vi "采集的条码数组.vi"(9 "条码数量":i32, 10 "地址":string, 11 "开启条码?":bool) -> (1 "条码字符串":string, 2 "条码数组":string[](array[string]), 3 "料号":string[](array[string]))   [LabVIEW 2014]
panel:
  out "数组":string[](array[string])
  out "数据输出":string
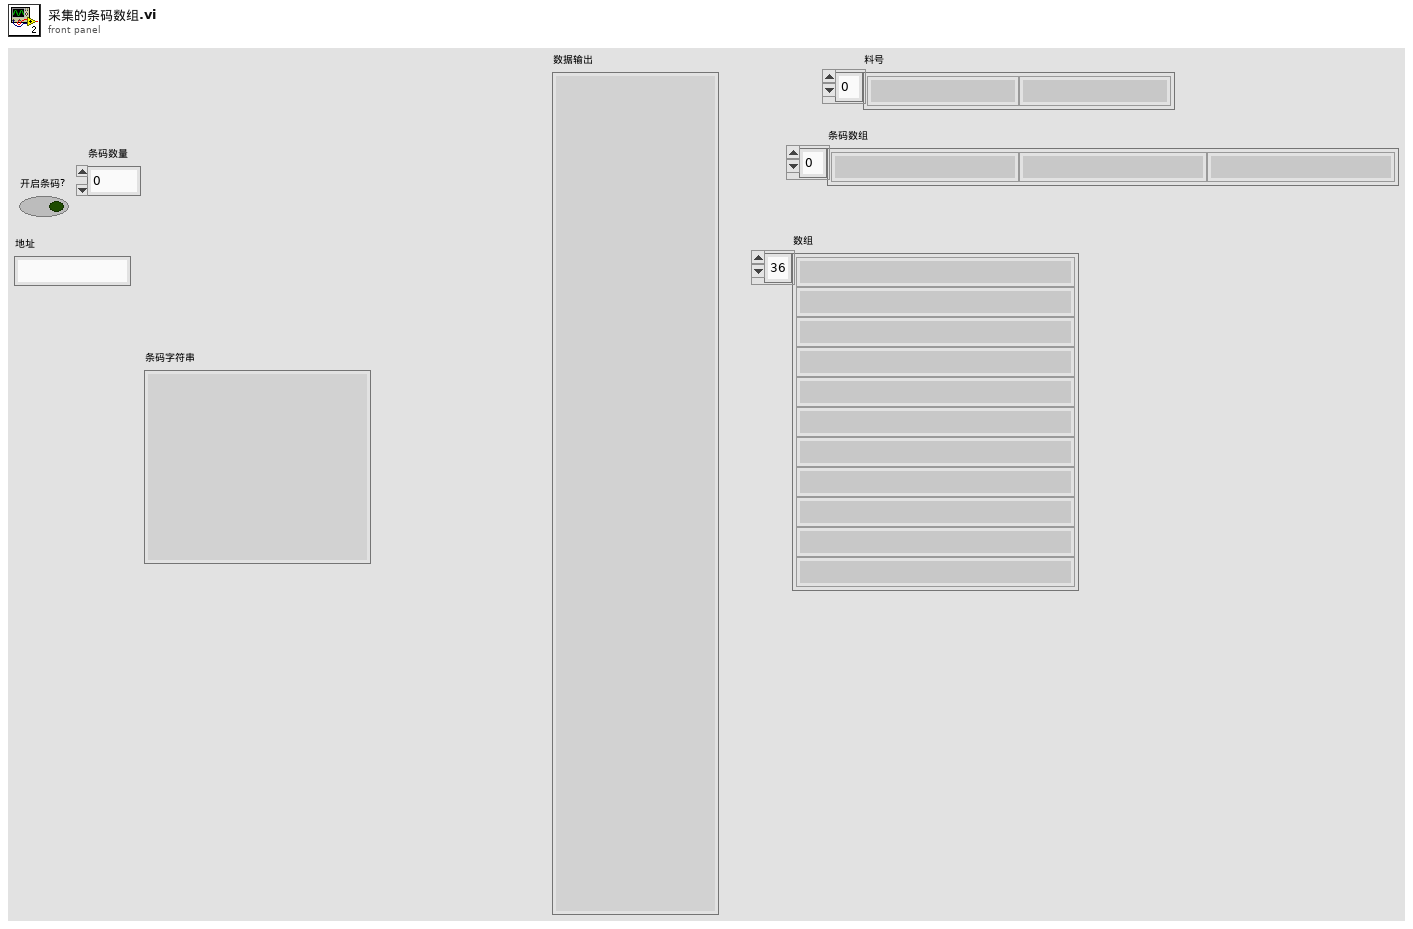
[diagram p1: front panel]
types:
  T1 = enum16{"Standard", "Buffered", "CRLF", "Immediate"}
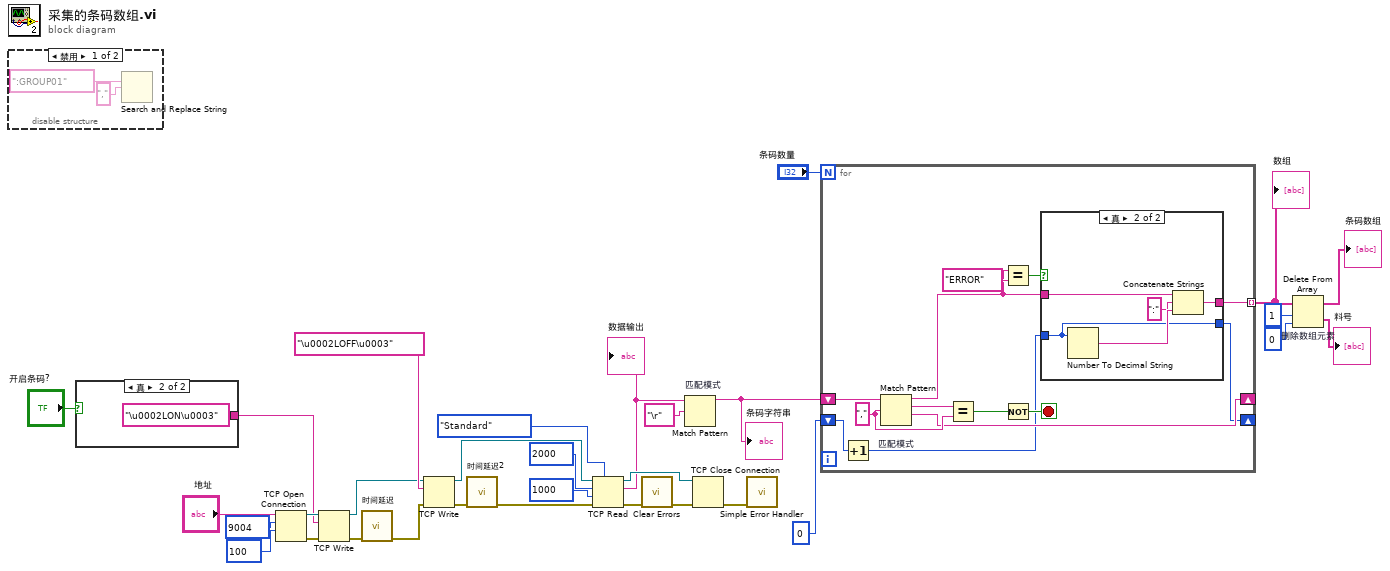
[diagram p0: block diagram]
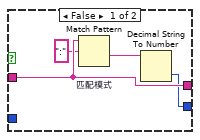
[diagram p3: hidden frame]
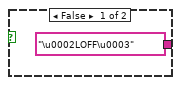
[diagram p4: hidden frame]
diagram:
  n1 = disable-structure shown="禁用" {
    frame Disabled {
      n2 = Search and Replace String ("搜索替换字符串")(search string=":GROUP01" ("正则表达式"), replace string="," ("替换字符串(\"\")")) -> ()  [unwired: 6 in, 4 out]
    }
    frame Enabled {
    }
  }
  n3 = case shown="真" "开启条码?" {
    tunnel: ["\u0002LOFF\u0003" "\u0002LON\u0003"] -> w17
    frame False {
    }
    frame True {
    }
  }
  n4 = TCP Open Connection(address="地址", remote port or service name=u16 9004 ("远程端口或服务名称"), timeout ms (60000)=100 ("超时毫秒(60000)")) -> (connection ID=w22:refnum<k5>, error out=w13:errorcluster)  [unwired: 2 in]
  n5 = TCP Write(connection ID=w22, data in=w17, error in (no error)=w13) -> (connection ID out=w27:refnum<k5>, error out=w29:errorcluster)  [unwired: 1 in, 1 out]
  n6 = call "时间延迟"("error in (no error)"=w29) -> ("error out"=w30:errorcluster)  [unwired: 10 in]
  n7 = TCP Write(connection ID=w27, data in="\u0002LOFF\u0003", error in (no error)=w30) -> (connection ID out=w31:refnum<k5>, error out=w8:errorcluster)  [unwired: 1 in, 1 out]
  n8 = call "时间延迟2"("error in (no error)"=w8) -> ("error out"=w7:errorcluster)  [unwired: 10 in]
  n9 = TCP Read(connection ID=w31, bytes to read=2000 ("读取的字节"), error in (no error)=w7, 7:T1."Standard" ("模式（标准）"), 9:1000 ("超时毫秒(25000)")) -> (connection ID out=w19:refnum<k5>, data out=w10:string, error out=w26:errorcluster)
  "数据输出" <- w10
  n10 = call <vilib>:"Clear Errors.vi"("error in (no error)"=w26) -> ("error out"=w20:errorcluster)  [unwired: 5 in, 1 out]
  n11 = Match Pattern "匹配模式"(string=w10, regular expression="\r" ("正则表达式")) -> (before substring=w6:string)  [unwired: 1 in, 3 out]
  "条码字符串" <- w6
  n12 = TCP Close Connection(connection ID=w19, error in (no error)=w20) -> (error out=w18:errorcluster)  [unwired: 1 in, 1 out]
  n13 = call <vilib>:"Simple Error Handler.vi"("error in (no error)"=w18) -> ()  [unwired: 4 in, 5 out]
  n14 = for {
    N: "条码数量" -> [_]
    tunnel: [w39] -> w5 mode=indexing
    shift-right: [w43] -> _
    shift-left: w6 -> [w48]
    shift-right: [w38] -> _
    shift-left: 0 -> [w37]
    stop <- w44 stop-if-true
    w45 = ","
    n15 = Increment(x=w37) -> (x+1=w36:i32)
    n16 = Match Pattern "匹配模式"(string=w48, regular expression=w45) -> (before substring=w40:string, match substring=w46:string, after substring=w43:string)  [unwired: 1 in, 1 out]
    n17 = Equal?(x=w46, y=w45) -> (x = y?=w47:bool)
    n18 = Equal?(x=w40, y="ERROR") -> (x = y?=w41:bool)
    n19 = Not(x=w47) -> (.not. x?=w44:bool)
    n20 = case shown="真" w41 {
      tunnel: [w52 w55] -> w39
      tunnel: w40 -> [w52 w57]
      tunnel: [w49 w54] -> w38
      tunnel: w36 -> [_ w54]
      frame False {
        n21 = Match Pattern "匹配模式"(string=w52, regular expression=":" ("正则表达式")) -> (after substring=w50:string)  [unwired: 1 in, 3 out]
        n22 = Decimal String To Number(string=w50) -> (number=w49:i32)  [unwired: 2 in, 1 out]
      }
      frame True {
        n23 = Number To Decimal String(number=w54) -> (decimal integer string=w56:string)  [unwired: 1 in]
        n24 = Concatenate Strings(w57, ":" ("字符串"), w56) -> (w55:string)
      }
    }
  }
  "数组" <- w5
  n25 = Delete From Array "删除数组元素"(array=w5, length=1 ("长度"), index=0 ("索引")) -> (deleted portion=→"料号":string[], array with subset deleted=→"条码数组":string[])
